vi "signalAccumulate randomData.vi"() -> (0 "Data":cluster{"X":dbl[], "Y":sgl[]}[](array[cluster]))   [LabVIEW 2018]
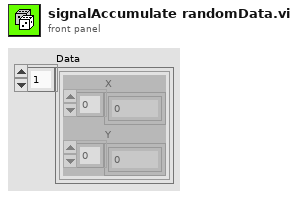
[diagram p1: front panel]
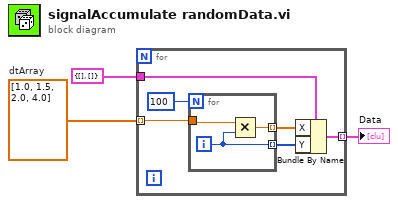
[diagram p0: block diagram]
diagram:
  w3 = dbl[] [1.0, 1.5, 2.0, 4.0]  # dtArray
  n1 = for {
    tunnel: w3 -> [w8] mode=indexing
    tunnel: cluster{"X":dbl[], "Y":sgl[]} {"X"=[], "Y"=[]} ("MassSpectrum") -> [w7]
    tunnel: [w4] -> w1 mode=indexing
    n2 = for {
      N: 100 -> [_]
      tunnel: [w12] -> w5 mode=indexing
      tunnel: w8 -> [w11]
      tunnel: [w10] -> w6 mode=indexing
      i -> [w12]
      n3 = Multiply(x=w11, y=w12) -> (x*y=w10:dbl)
    }
    n4 = Bundle By Name(cluster=w7, "X"=w6, "Y"=w5) -> (w4:cluster{"X":dbl[], "Y":sgl[]})
  }
  "Data" <- w1
